vi "LVClass_SlopesPostProcessList AddProcessor_Filter.vi"(0 "SlopesPostProcessorList in":refnum<class "SlopesPostProcessorList.lvclass">, 5 "Position":i32, 7 "Filter":T1, 11 "error in (no error)":errorcluster) -> (4 "SlopesPostProcessorList out":refnum<class "SlopesPostProcessorList.lvclass">, 15 "error out":errorcluster)   [LabVIEW 2020, in "SlopesPostProcessorList.lvclass"]
doc: "Insert a Filter processor.\n\n--------------------------------------------------------------------------------\n\n<B>SlopesPostProcessorListIn </B> : SlopesPostProcessorList object.\n<B>SlopesPostProcessorListOut </B> : SlopesPostProcessorList object.\n<B>position </B> : Position of the processor in the SlopesPostProcessorList.\n<B>apply_tiltx_filter </B> : Activate x tilt filter.\n<B>apply_tilty_filter </B> : Activate y tilt filter.\n<B>apply_curv_filter </B> : Activate curvature filter.\n<B>apply_astig0_filter </B> : Activate 0 degree astigmatism filter.\n<B>apply_astig45_filter </B> : Activate 45 degree astigmatism filter.\n<B>apply_others_filter </B> : Activate all other aberrations filter.\n<B>ErrorIn </B> : Error\n<B>ErrorOut </B> : Error\n\n--------------------------------------------------------------------------------"
uses:
  SlopesPostProcessorList.lvclass
  Controls/SlopesPostProcessorList - Filter.ctl
  SlopesPostProcessorList.lvclass/SlopesPostProcessorList.ctl
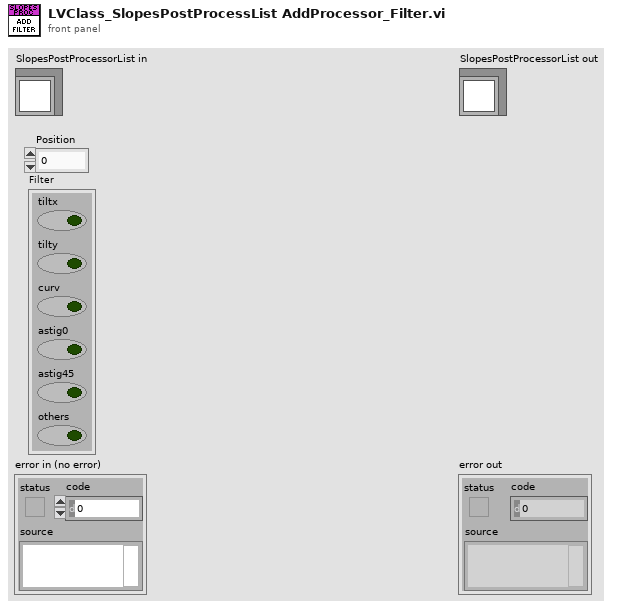
[diagram p1: front panel]
types:
  T1 = typedef "SlopesPostProcessorList - Filter.ctl" = cluster{"tiltx":bool, "tilty":bool, "curv":bool, "astig0":bool, "astig45":bool, "others":bool}
  T2 = typedef "ClassID.ctl" = i64
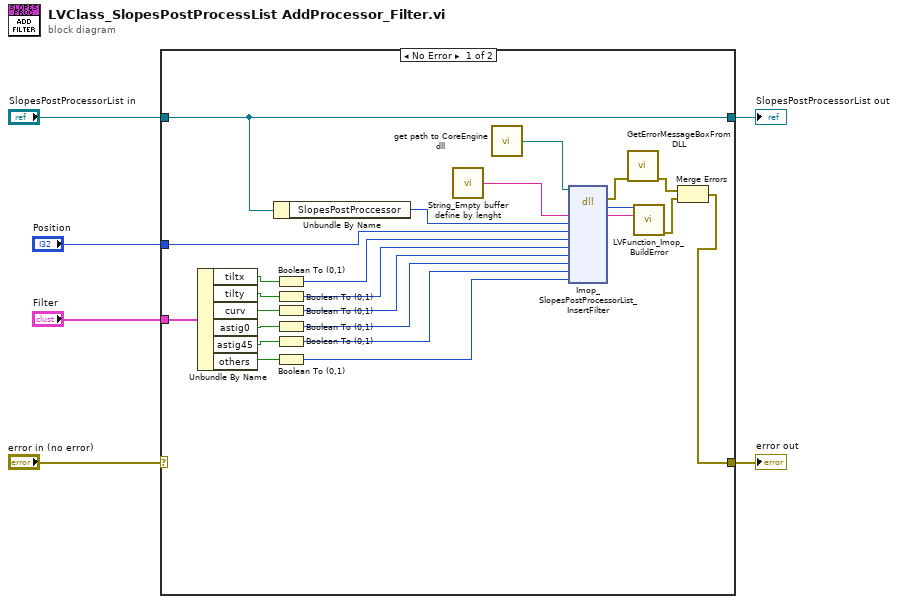
[diagram p0: block diagram]
diagram:
  n1 = case shown="No Error" "error in (no error)" {
    selector: "error in (no error)" -> [_ w32]
    tunnel: [w10 w32] -> w5
    tunnel: [w20 w31] -> w3
    tunnel: "SlopesPostProcessorList in" -> [w20 w31]
    tunnel: "Filter" -> [w18 _]
    tunnel: "Position" -> [w7 _]
    frame No Error {
      n2 = Unbundle By Name(w18) -> ("tiltx"=w17:bool, "tilty"=w16:bool, "curv"=w15:bool, "astig0"=w14:bool, "astig45"=w13:bool, "others"=w9:bool)
      n3 = Unbundle By Name(w20) -> ("SlopesPostProccessor"=w19:T2)
      n4 = Boolean To (0,1)(Boolean=w17) -> (0, 1=w25:i16)
      n5 = Boolean To (0,1)(Boolean=w16) -> (0, 1=w24:i16)
      n6 = Boolean To (0,1)(Boolean=w15) -> (0, 1=w23:i16)
      n7 = Boolean To (0,1)(Boolean=w14) -> (0, 1=w22:i16)
      n8 = Boolean To (0,1)(Boolean=w13) -> (0, 1=w21:i16)
      n9 = Boolean To (0,1)(Boolean=w9) -> (0, 1=w8:i16)
      n10 = call "String_Empty buffer define by lenght.vi"() -> ("Empty buffer"=w30:string)  [unwired: 1 in]
      n11 = call "get path to CoreEngine dll.vi"() -> ("path to wavekit library"=w27:path)  [unwired: 14 in, 1 out]
      n12 = dll-call lib="D:/soft/HASO_v3/SVN_trunk/ImOpCoreEngine4_LV2011/DLLs/c_interface_vc100.dll" fn="Imop_SlopesPostProcessorList_InsertFilter"(path in=w27, "message"=w30, "objet"=w19, "Position"=w7, "tiltX"=w25, "tiltY"=w24, "Curv"=w23, "Astig0"=w22, "Astig45"=w21, "others"=w8) -> (error out=w26:errorcluster, "return type"=w28:i32, "message"=w29:string)  [unwired: 10 in, 1 out]
      n13 = call "GetErrorMessageBoxFromDLL.vi"("error IN"=w26) -> ("error OUT"=w12:errorcluster)  [unwired: 10 in]
      n14 = call "LVFunction_Imop_BuildError.vi"("code"=w28, "String to Prepend to source (\"\")"=w29) -> ("error out"=w11:errorcluster)  [unwired: 13 in]
      n15 = Merge Errors(w12, w11) -> (w10:errorcluster)
    }
    frame Error {
    }
  }
  "error out" <- w5
  "SlopesPostProcessorList out" <- w3
